vi "ex_getDaqmxChannelProperties.vi"(4 "error in (no error)":errorcluster, 5 "USI compliant names":bool, 6 "Number of channels (if no DAQmx task available)":i32, 7 "task":T4) -> (0 "error out":errorcluster, 1 "all properties":T1, 3 "channel properties":T2[][](array[typedef]))   [LabVIEW 2017]
uses:
  <vilib>/express/express shared/ex_EditUserDefinedProperties/ex_userdefproperties.ctl
  <vilib>/express/express shared/ExFile.llb/ex_userDefProperty.ctl
  <vilib>/express/express shared/ex_EditUserDefinedProperties/usiDataType.ctl
  <vilib>/express/express shared/ExFile.llb/ex_propertySource.ctl
  <vilib>/express/express shared/ExFile.llb/ex_TdmProperty.ctl
  <vilib>/express/express shared/ExFile.llb/ex_TdmData.ctl
panel:
  in  "File data":T1
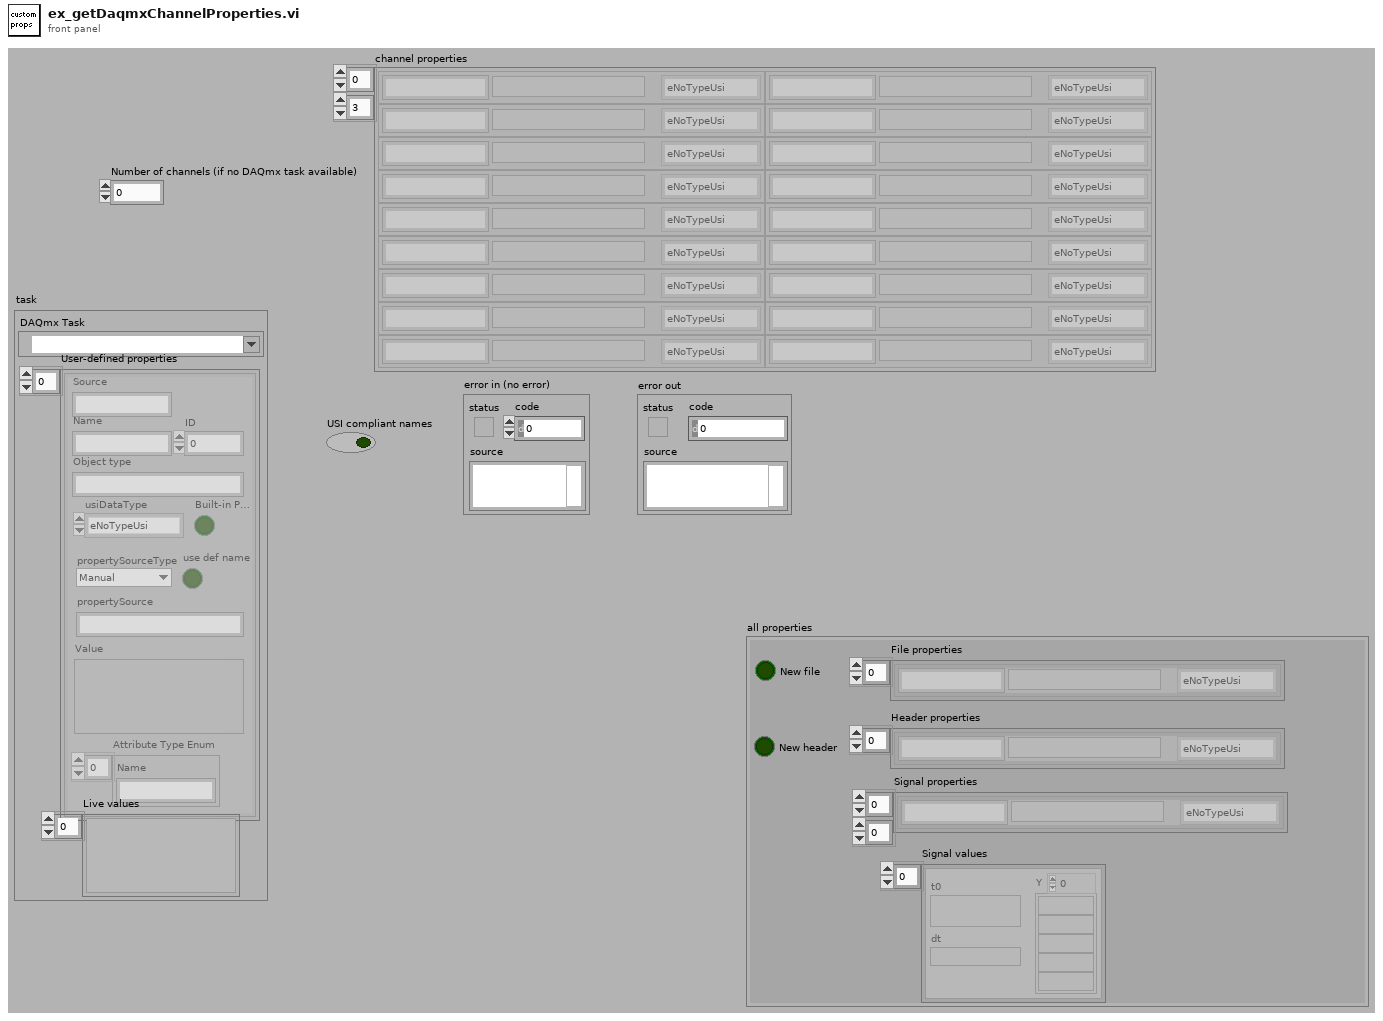
[diagram p1: front panel]
types:
  T1 = typedef "ex_TdmData.ctl" = cluster{"New file":bool, "New header":bool, "File properties":T2[], "Header properties":T2[], "Signal properties":T2[][], "Signal values":waveform(dbl)[]}
  T2 = typedef "ex_TdmProperty.ctl" = cluster{"Name":string, "Type":T3, "Value":variant}
  T3 = typedef "usiDataType.ctl" = enum16{"eNoTypeUsi", "eInt8Usi", "eInt16Usi", "eInt32Usi", "eInt64Usi", "eUInt8Usi", "eUInt16Usi", "eUInt32Usi", "eUInt64Usi", "eFloat32Usi", "eFloat64Usi", "- 0", "- 1", "- 2", "- 3", "- 4", "- 5", "- 6", "- 7", "- 8", "- 9", "eString8Usi", "eString16Usi", "eStringUsi", "eEnumUsi", "- 10", "- 11", "- 12", "- 13", "- 14", "eTimeUsi", "- 15", "- 16", "- 17", "- 18", "- 19", "- 20", "- 21", "- 22", "- 23", "eInstanceUsi", "eStoreUsi"}
  T4 = typedef "ex_userdefproperties.ctl" = cluster{"DAQmx Task":refnum<k21>, "User-defined properties":T5[], "Live values":variant[]}
  T5 = typedef "ex_userDefProperty.ctl" = cluster{"Name":string, "Object type":string, "usiDataType":T3, "propertySourceType":T6, "propertySource":string, "Value":variant, "ID":i32, "use def name":bool, "Source":string, "Built-in Prop":bool, "Attribute Type Enum":string[]}
  T6 = typedef "ex_propertySource.ctl" = enum16{"Manual", "System", "DAQmx Channel", "Terminal", "Ignore"}
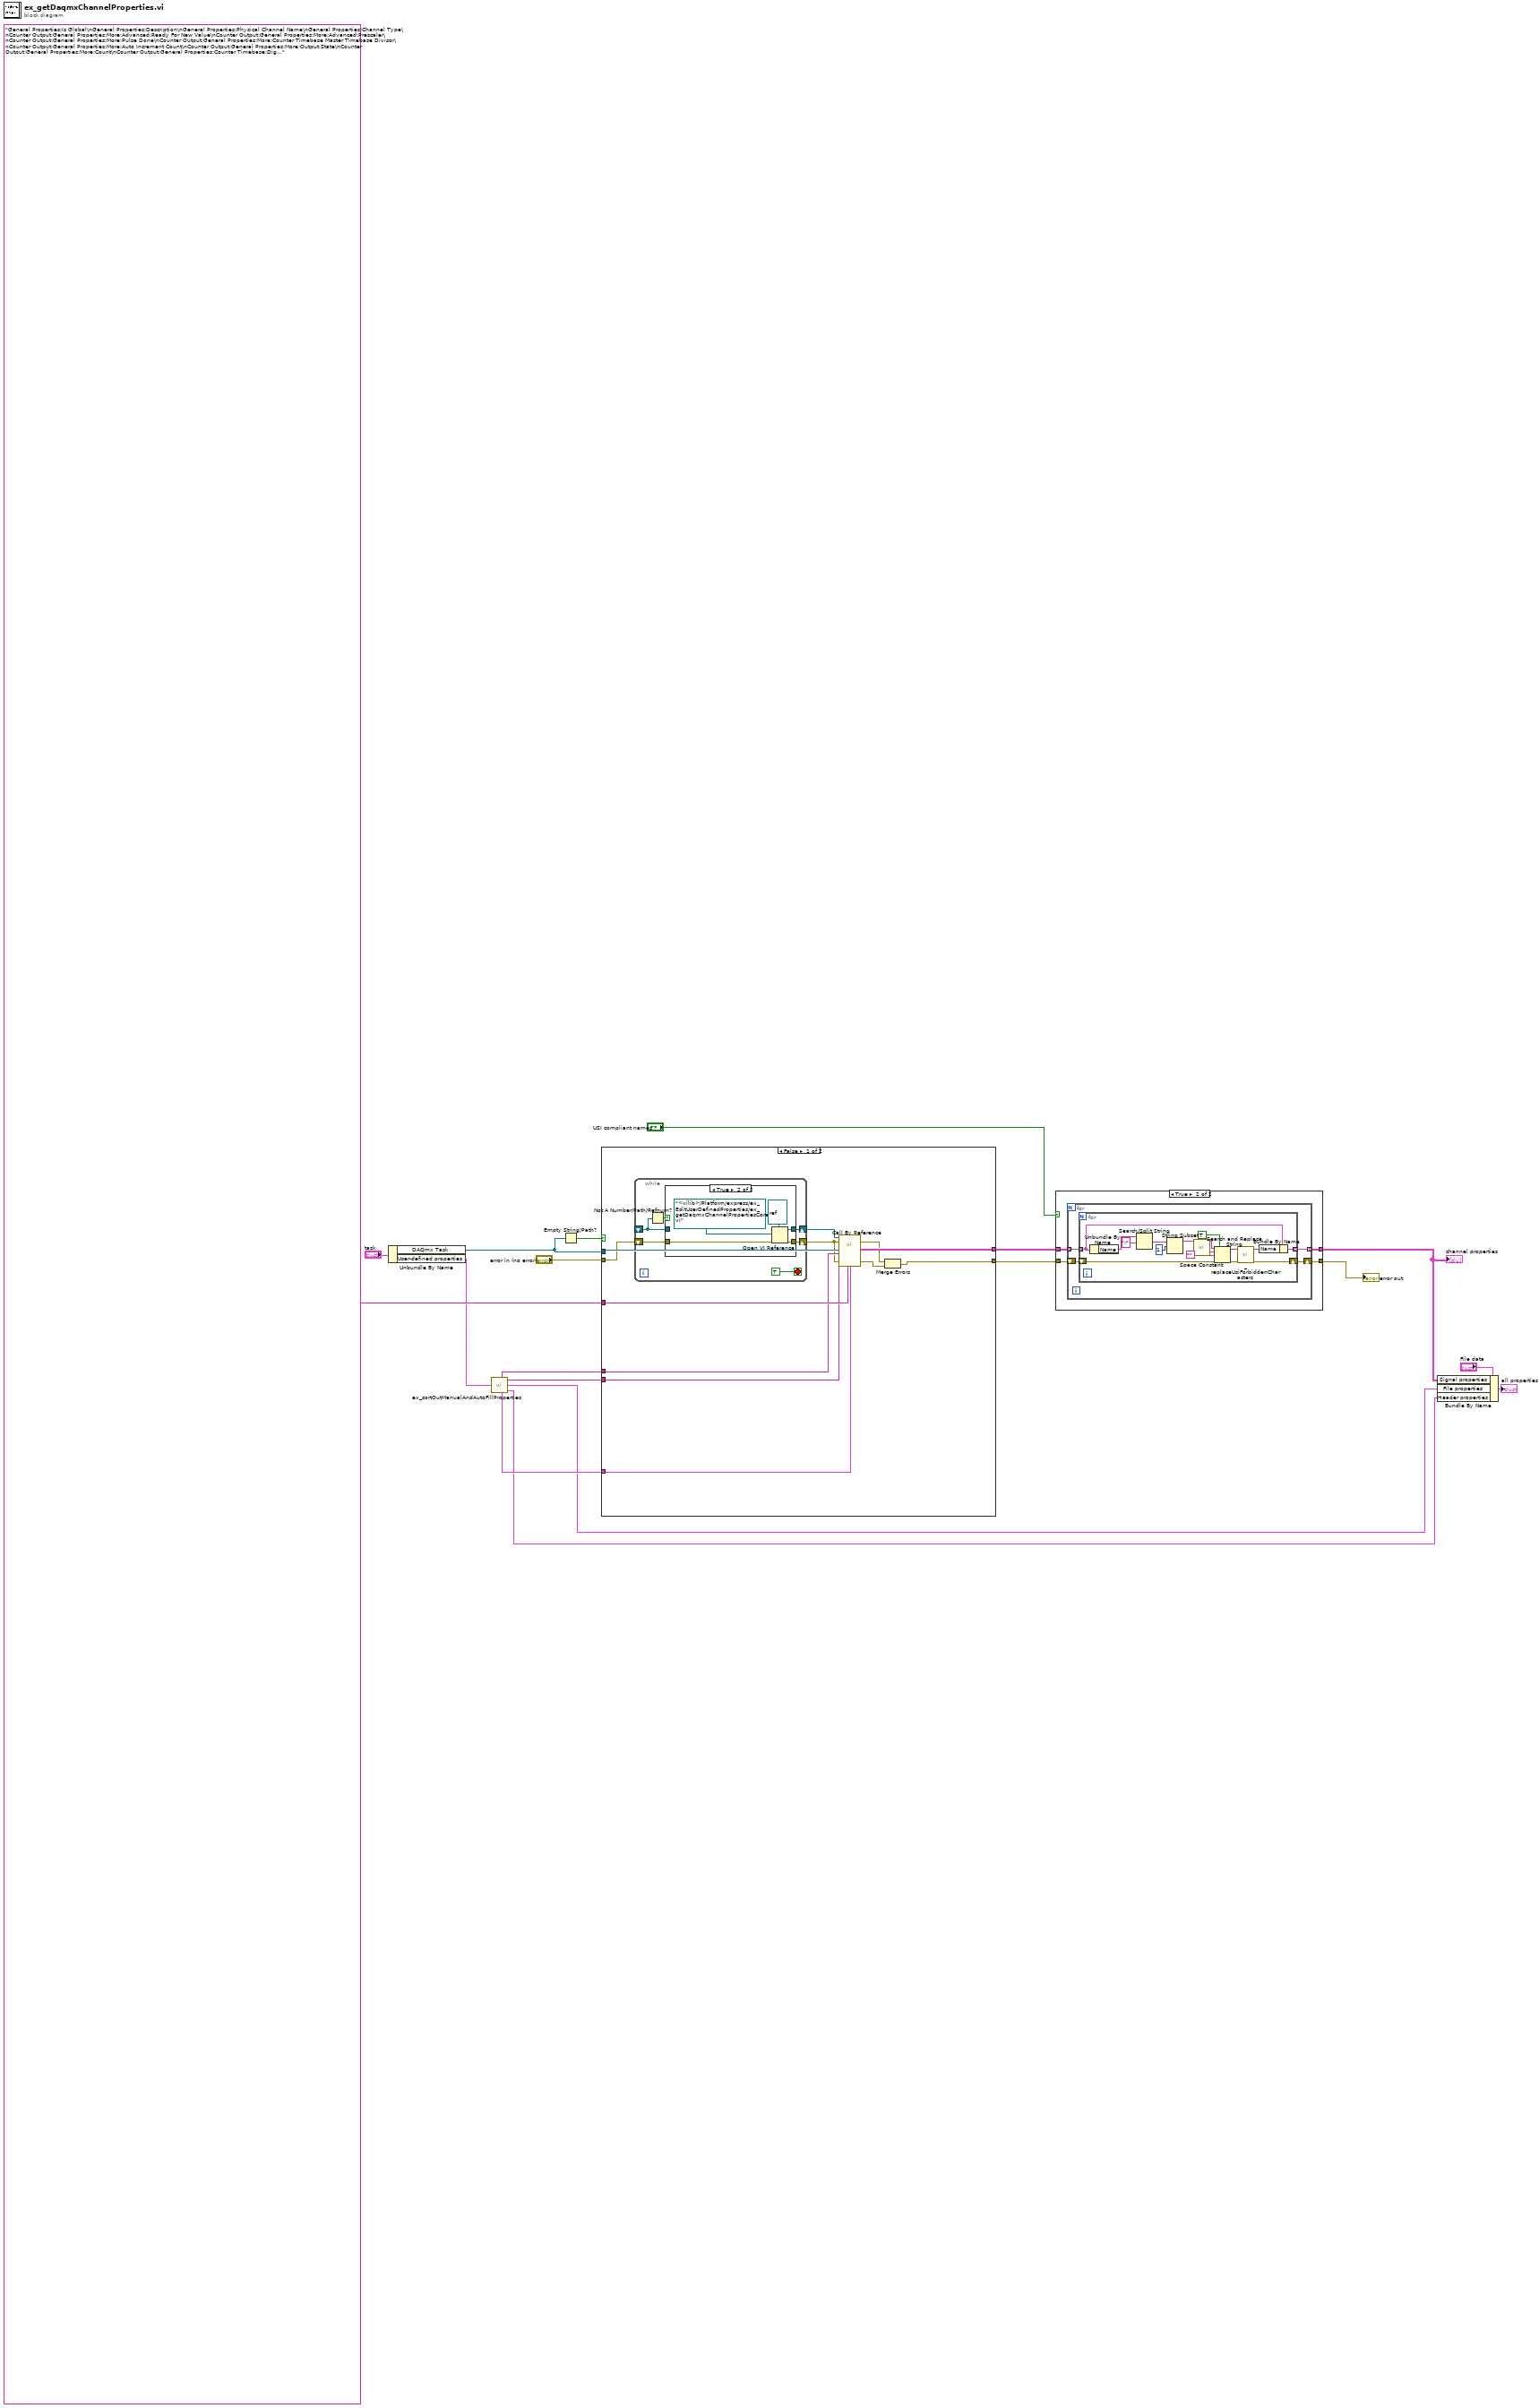
[diagram p0: block diagram]
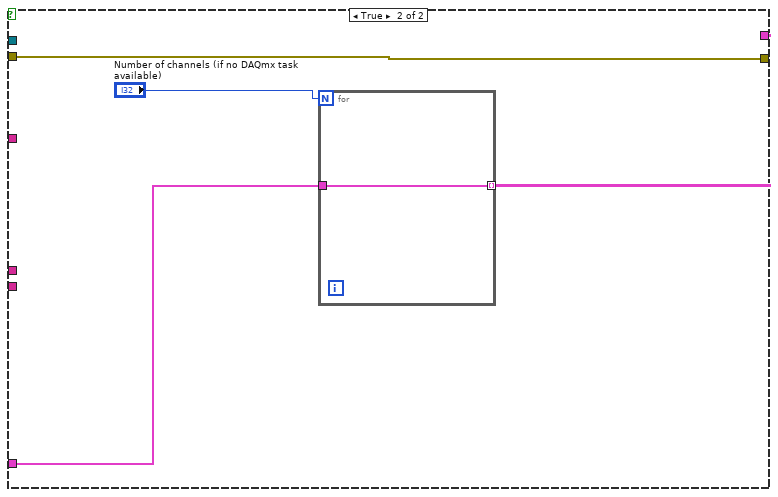
[diagram p3: hidden frame]
diagram:
  n1 = Unbundle By Name("task") -> ("DAQmx Task"=w2:refnum<k21>, "User-defined properties"=w13:T5[])
  n2 = call <vilib>:"ex_sortOutManualAndAutoFillProperties.vi"("User-defined properties"=w13) -> ("channelgroup props"=w6:T2[], "channel props"=w10:T2[], "file props"=w7:T2[], "property names (manual)"=w12:string[], "property names (autofill)"=w11:string[])
  n3 = Empty String/Path?(string/path=w2) -> (empty?=w1:bool)
  n4 = case shown="False" w1 {
    tunnel: "General Properties:Is Global\nGeneral Properties:Description\nGeneral Properties:Physical Channel Name\nGeneral Properties:Channel Type\nCounter Output:General Properties:More:Advanced:Ready For New Value\nCounter Output:General Properties:More:Advanced:Prescaler\nCounter Output:General Properties:More:Pulse Done\nCounter Output:General Properties:More:Counter Timebase Master Timebase Divisor\nCounter Output:General Properties:More:Auto Increment Count\nCounter Output:General Properties:More:Output State\nCounter Output:General Properties:More:Count\nCounter Output:General Properties:Counter Timebase:Digital Synchronization:Enable\nCounter Output:General Properties:Counter Timebase:Digital Filter:Timebase:Rate\nCounter Output:General Properties:Counter Timebase:Digital Filter:Timebase:Source\nCounter Output:General Properties:Counter Timebase:Digital Filter:Minimum Pulse Width\nCounter Output:General Properties:Counter Timebase:Digital Filter:Enable\nCounter Output:General Properties:Counter Timebase:Active Edge\nCounter Output:General Properties:Counter Timebase:Rate\nCounter Output:General Properties:Counter Timebase:Source\nCounter Output:Pulse:Ticks:Initial Delay\nCounter Output:Pulse:Ticks:Low Ticks\nCounter Output:Pulse:Ticks:High Ticks\nCounter Output:Pulse:Frequency:Initial Delay\nCounter Output:Pulse:Frequency:Frequency\nCounter Output:Pulse:Frequency:Units\nCounter Output:Pulse:Frequency:Duty Cycle\nCounter Output:Pulse:Time:Initial Delay\nCounter Output:Pulse:Time:Low Time\nCounter Output:Pulse:Time:High Time\nCounter Output:Pulse:Time:Units\nCounter Output:Pulse:Output Terminal\nCounter Output:Pulse:Idle State\nCounter Output:Output Type\nCounter Input:General Properties:More:Advanced:Prescaler\nCounter Input:General Properties:More:Advanced:Duplicate Count Prevention\nCounter Input:General Properties:More:Advanced:Data Transfer and Memory:Number Of Possibly Invalid Samples\nCounter Input:General Properties:More:Advanced:Data Transfer and Memory:Data Transfer Mechanism\nCounter Input:General Properties:More:Counter Timebase Master Timebase Divisor\nCounter Input:General Properties:More:Terminal Count Reached\nCounter Input:General Properties:More:Output State\nCounter Input:General Properties:More:Count\nCounter Input:General Properties:Counter Timebase:Digital Synchronization:Enable\nCounter Input:General Properties:Counter Timebase:Digital Filter:Timebase:Rate\nCounter Input:General Properties:Counter Timebase:Digital Filter:Timebase:Source\nCounter Input:General Properties:Counter Timebase:Digital Filter:Minimum Pulse Width\nCounter Input:General Properties:Counter Timebase:Digital Filter:Enable\nCounter Input:General Properties:Counter Timebase:Active Edge\nCounter Input:General Properties:Counter Timebase:Rate\nCounter Input:General Properties:Counter Timebase:Source\nCounter Input:Timestamp:GPS:Synchronization Source\nCounter Input:Timestamp:GPS:Synchronization Method\nCounter Input:Timestamp:Initial Seconds\nCounter Input:Timestamp:Units\nCounter Input:Semi-Period:Digital Synchronization:Enable\nCounter Input:Semi-Period:Digital Filter:Timebase:Rate\nCounter Input:Semi-Period:Digital Filter:Timebase:Source\nCounter Input:Semi-Period:Digital Filter:Minimum Pulse Width\nCounter Input:Semi-Period:Digital Filter:Enable\nCounter Input:Semi-Period:Starting Edge\nCounter Input:Semi-Period:Input Terminal\nCounter Input:Semi-Period:Units\nCounter Input:Two Edge Separation:Second:Digital Synchronization:Enable\nCounter Input:Two Edge Separation:Second:Digital Filter:Timebase:Rate\nCounter Input:Two Edge Separation:Second:Digital Filter:Timebase:Source\nCounter Input:Two Edge Separation:Second:Digital Filter:Minimum Pulse Width\nCounter Input:Two Edge Separation:Second:Digital Filter:Enable\nCounter Input:Two Edge Separation:Second:Edge\nCounter Input:Two Edge Separation:Second:Input Terminal\nCounter Input:Two Edge Separation:First:Digital Synchronization:Enable\nCounter Input:Two Edge Separation:First:Digital Filter:Timebase:Rate\nCounter Input:Two Edge Separation:First:Digital Filter:Timebase:Source\nCounter Input:Two Edge Separation:First:Digital Filter:Minimum Pulse Width\nCounter Input:Two Edge Separation:First:Digital Filter:Enable\nCounter Input:Two Edge Separation:First:Edge\nCounter Input:Two Edge Separation:First:Input Terminal\nCounter Input:Two Edge Separation:Units\nCounter Input:Pulse Width:Digital Synchronization:Enable\nCounter Input:Pulse Width:Digital Filter:Timebase:Rate\nCounter Input:Pulse Width:Digital Filter:Timebase:Source\nCounter Input:Pulse Width:Digital Filter:Minimum Pulse Width\nCounter Input:Pulse Width:Digital Filter:Enable\nCounter Input:Pulse Width:Starting Edge\nCounter Input:Pulse Width:Input Terminal\nCounter Input:Pulse Width:Units\nCounter Input:Position:Z Index Phase\nCounter Input:Position:Z Index Value\nCounter Input:Position:Z Index Enable\nCounter Input:Position:Z Input:Digital Synchronization:Enable\nCounter Input:Position:Z Input:Digital Filter:Timebase:Rate\nCounter Input:Position:Z Input:Digital Filter:Timebase:Source\nCounter Input:Position:Z Input:Digital Filter:Minimum Pulse Width\nCounter Input:Position:Z Input:Digital Filter:Enable\nCounter Input:Position:Z Input:Terminal\nCounter Input:Position:B Input:Digital Synchronization:Enable\nCounter Input:Position:B Input:Digital Filter:Timebase:Rate\nCounter Input:Position:B Input:Digital Filter:Timebase:Source\nCounter Input:Position:B Input:Digital Filter:Minimum Pulse Width\nCounter Input:Position:B Input:Digital Filter:Enable\nCounter Input:Position:B Input:Terminal\nCounter Input:Position:A Input:Digital Synchronization:Enable\nCounter Input:Position:A Input:Digital Filter:Timebase:Rate\nCounter Input:Position:A Input:Digital Filter:Timebase:Source\nCounter Input:Position:A Input:Digital Filter:Minimum Pulse Width\nCounter Input:Position:A Input:Digital Filter:Enable\nCounter Input:Position:A Input:Terminal\nCounter Input:Position:Decoding Type\nCounter Input:Position:Linear Encoder:Initial Position\nCounter Input:Position:Linear Encoder:Distance Per Pulse\nCounter Input:Position:Linear Encoder:Units\nCounter Input:Position:Angular Encoder:Initial Angle\nCounter Input:Position:Angular Encoder:Pulses Per Revolution\nCounter Input:Position:Angular Encoder:Units\nCounter Input:Count Edges:Digital Synchronization:Enable\nCounter Input:Count Edges:Digital Filter:Timebase:Rate\nCounter Input:Count Edges:Digital Filter:Timebase:Source\nCounter Input:Count Edges:Digital Filter:Minimum Pulse Width\nCounter Input:Count Edges:Digital Filter:Enable\nCounter Input:Count Edges:Active Edge\nCounter Input:Count Edges:Initial Count\nCounter Input:Count Edges:Count Direction:Digital Synchronization:Enable\nCounter Input:Count Edges:Count Direction:Digital Filter:Timebase:Rate\nCounter Input:Count Edges:Count Direction:Digital Filter:Timebase:Source\nCounter Input:Count Edges:Count Direction:Digital Filter:Minimum Pulse Width\nCounter Input:Count Edges:Count Direction:Digital Filter:Enable\nCounter Input:Count Edges:Count Direction:Terminal\nCounter Input:Count Edges:Count Direction:Direction\nCounter Input:Count Edges:Input Terminal\nCounter Input:Period:Digital Synchronization:Enable\nCounter Input:Period:Digital Filter:Timebase:Rate\nCounter Input:Period:Digital Filter:Timebase:Source\nCounter Input:Period:Digital Filter:Minimum Pulse Width\nCounter Input:Period:Digital Filter:Enable\nCounter Input:Period:Measurement Specifications:Large Range:Divisor\nCounter Input:Period:Measurement Specifications:High Frequency:Measurement Time\nCounter Input:Period:Measurement Specifications:Method\nCounter Input:Period:Starting Edge\nCounter Input:Period:Input Terminal\nCounter Input:Period:Units\nCounter Input:Frequency:Digital Synchronization:Enable\nCounter Input:Frequency:Digital Filter:Timebase:Rate\nCounter Input:Frequency:Digital Filter:Timebase:Source\nCounter Input:Frequency:Digital Filter:Minimum Pulse Width\nCounter Input:Frequency:Digital Filter:Enable\nCounter Input:Frequency:Measurement Specifications:Large Range:Divisor\nCounter Input:Frequency:Measurement Specifications:High Frequency:Measurement Time\nCounter Input:Frequency:Measurement Specifications:Method\nCounter Input:Frequency:Starting Edge\nCounter Input:Frequency:Input Terminal\nCounter Input:Frequency:Units\nCounter Input:Measurement Type\nCounter Input:Custom Scale Name\nCounter Input:Minimum Value\nCounter Input:Maximum Value\nDigital Output:General Properties:Advanced:Data Transfer and Memory:Data Transfer Request Condition\nDigital Output:General Properties:Advanced:Data Transfer and Memory:Data Transfer Mechanism\nDigital Output:General Properties:Advanced:Data Transfer and Memory:Use Only Onboard Memory\nDigital Output:Tristate\nDigital Output:Number of Lines\nDigital Output:Invert Lines\nDigital Output:Output Drive Type\nDigital Input:General Properties:Advanced:Data Transfer and Memory:Data Transfer Request Condition\nDigital Input:General Properties:Advanced:Data Transfer and Memory:Data Transfer Mechanism\nDigital Input:Tristate\nDigital Input:Digital Filter:Minimum Pulse Width\nDigital Input:Digital Filter:Enable\nDigital Input:Number of Lines\nDigital Input:Invert Lines\nAnalog Output:General Properties:Advanced:Enhanced Image Rejection Enable\nAnalog Output:General Properties:Advanced:Device Scaling Coefficients:Device Scaling Coefficients\nAnalog Output:General Properties:Advanced:Data Transfer and Memory:Memory Mapping for Programmed IO Enable\nAnalog Output:General Properties:Advanced:Data Transfer and Memory:Data Transfer Request Condition\nAnalog Output:General Properties:Advanced:Data Transfer and Memory:Data Transfer Mechanism\nAnalog Output:General Properties:Advanced:Data Transfer and Memory:Use Only Onboard Memory\nAnalog Output:General Properties:Advanced:Gain:Gain Value\nAnalog Output:General Properties:DAC:Reglitching Enable\nAnalog Output:General Properties:DAC:Offset Voltage:Value\nAnalog Output:General Properties:DAC:Offset Voltage:External Source\nAnalog Output:General Properties:DAC:Offset Voltage:Source\nAnalog Output:General Properties:DAC:Reference Voltage:Value\nAnalog Output:General Properties:DAC:Reference Voltage:External Source\nAnalog Output:General Properties:DAC:Reference Voltage:Source\nAnalog Output:General Properties:DAC:Reference Voltage:Allow Connecting DAC Reference to Ground at Runtime\nAnalog Output:General Properties:DAC:Reference Voltage:Connect DAC Reference to Ground\nAnalog Output:General Properties:DAC:Range:Low\nAnalog Output:General Properties:DAC:Range:High\nAnalog Output:General Properties:DAC:Resolution Value\nAnalog Output:General Properties:DAC:Resolution Units\nAnalog Output:General Properties:Output Configuration:Terminal Configuration\nAnalog Output:General Properties:Output Configuration:Idle Output Behavior\nAnalog Output:General Properties:Output Configuration:Load Impedance\nAnalog Output:General Properties:Output Configuration:Output Impedance\nAnalog Output:Current:Units\nAnalog Output:Voltage:Units\nAnalog Output:Output Type\nAnalog Output:Custom Scale Name\nAnalog Output:Minimum Value\nAnalog Output:Maximum Value\nAnalog Input:General Properties:Advanced:Enhanced Alias Rejection Enable\nAnalog Input:General Properties:Advanced:Device Scaling Coefficients:Device Scaling Coefficients\nAnalog Input:General Properties:Advanced:Data Transfer and Memory:Compression:Lossy LSB Removal:Compressed Sample Size\nAnalog Input:General Properties:Advanced:Data Transfer and Memory:Compression:Raw Data Compression Type\nAnalog Input:General Properties:Advanced:Data Transfer and Memory:Memory Mapping for Programmed IO Enable\nAnalog Input:General Properties:Advanced:Data Transfer and Memory:Data Transfer Custom Threshold\nAnalog Input:General Properties:Advanced:Data Transfer and Memory:Data Transfer Request Condition\nAnalog Input:General Properties:Advanced:Data Transfer and Memory:Data Transfer Mechanism\nAnalog Input:General Properties:Advanced:High Accuracy Settings:Auto Zero Mode\nAnalog Input:General Properties:Advanced:Sample and Hold Enable\nAnalog Input:General Properties:Advanced:Gain:Gain Value\nAnalog Input:General Properties:Advanced:Range:Low\nAnalog Input:General Properties:Advanced:Range:High\nAnalog Input:General Properties:Channel Calibration:Verification:Acquired Values\nAnalog Input:General Properties:Channel Calibration:Verification:Reference Values\nAnalog Input:General Properties:Channel Calibration:Description\nAnalog Input:General Properties:Channel Calibration:Operator Name\nAnalog Input:General Properties:Channel Calibration:Scaling Parameters:Polynomial:Reverse Coefficients\nAnalog Input:General Properties:Channel Calibration:Scaling Parameters:Polynomial:Forward Coefficients\nAnalog Input:General Properties:Channel Calibration:Scaling Parameters:Table:Scaled Values\nAnalog Input:General Properties:Channel Calibration:Scaling Parameters:Table:Pre-Scaled Values\nAnalog Input:General Properties:Channel Calibration:Scaling Parameters:Scale Type\nAnalog Input:General Properties:Channel Calibration:Expiration Date\nAnalog Input:General Properties:Channel Calibration:Calibration Date\nAnalog Input:General Properties:Channel Calibration:Apply Calibration If Expired\nAnalog Input:General Properties:Channel Calibration:Enable Calibration\nAnalog Input:General Properties:Channel Calibration:Has Valid Calibration Information\nAnalog Input:General Properties:Digitizer/ADC:Dither:Enable\nAnalog Input:General Properties:Digitizer/ADC:Raw Sample Justification\nAnalog Input:General Properties:Digitizer/ADC:Raw Sample Size\nAnalog Input:General Properties:Digitizer/ADC:Resolution Value\nAnalog Input:General Properties:Digitizer/ADC:Resolution Units\nAnalog Input:General Properties:Filter:Analog Lowpass:Advanced:Switched Capacitor:Output Clock Divisor\nAnalog Input:General Properties:Filter:Analog Lowpass:Advanced:Switched Capacitor:External Clock Divisor\nAnalog Input:General Properties:Filter:Analog Lowpass:Advanced:Switched Capacitor:External Clock Frequency\nAnalog Input:General Properties:Filter:Analog Lowpass:Advanced:Switched Capacitor:Clock Source\nAnalog Input:General Properties:Filter:Analog Lowpass:Cutoff Frequency\nAnalog Input:General Properties:Filter:Analog Lowpass:Enable\nAnalog Input:General Properties:Signal Conditioning:Probe/Attenuator:Attenuation Value\nAnalog Input:General Properties:Signal Conditioning:Excitation:AC Excitation:Wire Mode\nAnalog Input:General Properties:Signal Conditioning:Excitation:AC Excitation:Synchronization Enable\nAnalog Input:General Properties:Signal Conditioning:Excitation:AC Excitation:Frequency\nAnalog Input:General Properties:Signal Conditioning:Excitation:Advanced:Voltage or Current\nAnalog Input:General Properties:Signal Conditioning:Excitation:Advanced:DC or AC\nAnalog Input:General Properties:Signal Conditioning:Excitation:Advanced:Actual Excitation Value\nAnalog Input:General Properties:Signal Conditioning:Excitation:Advanced:Use Multiplexed Excitation\nAnalog Input:General Properties:Signal Conditioning:Excitation:Advanced:Use Excitation For Scaling\nAnalog Input:General Properties:Signal Conditioning:Excitation:Value\nAnalog Input:General Properties:Signal Conditioning:Excitation:Source\nAnalog Input:General Properties:Signal Conditioning:Current Shunt Resistor:Value\nAnalog Input:General Properties:Signal Conditioning:Current Shunt Resistor:Location\nAnalog Input:General Properties:Signal Conditioning:Bridge:Balance:Fine Potentiometer\nAnalog Input:General Properties:Signal Conditioning:Bridge:Balance:Coarse Potentiometer\nAnalog Input:General Properties:Signal Conditioning:Bridge:Shunt Cal:Gain Adjustment\nAnalog Input:General Properties:Signal Conditioning:Bridge:Shunt Cal:Shunt Cal Select\nAnalog Input:General Properties:Signal Conditioning:Bridge:Shunt Cal:Shunt Cal Enable\nAnalog Input:General Properties:Signal Conditioning:Bridge:Initial Bridge Voltage\nAnalog Input:General Properties:Signal Conditioning:Bridge:Nominal Resistance\nAnalog Input:General Properties:Signal Conditioning:Bridge:Configuration\nAnalog Input:General Properties:Signal Conditioning:Lead Wire Resistance\nAnalog Input:General Properties:Signal Conditioning:Resistance Configuration\nAnalog Input:General Properties:Input Configuration:Input Source\nAnalog Input:General Properties:Input Configuration:Terminal Configuration\nAnalog Input:General Properties:Input Configuration:Impedance\nAnalog Input:General Properties:Input Configuration:Coupling\nAnalog Input:TEDS:Units\nAnalog Input:Acceleration:Accelerometer:Sensitivity Units\nAnalog Input:Acceleration:Accelerometer:Sensitivity\nAnalog Input:Acceleration:Units\nAnalog Input:Sound Pressure:Microphone:Sensitivity\nAnalog Input:Sound Pressure:Units\nAnalog Input:Sound Pressure:Maximum Sound Pressure Level\nAnalog Input:Position:RVDT:Sensitivity Units\nAnalog Input:Position:RVDT:Sensitivity\nAnalog Input:Position:RVDT:Units\nAnalog Input:Position:LVDT:Sensitivity Units\nAnalog Input:Position:LVDT:Sensitivity\nAnalog Input:Position:LVDT:Units\nAnalog Input:Frequency:Voltage:Hysteresis\nAnalog Input:Frequency:Voltage:Threshold Level\nAnalog Input:Frequency:Units\nAnalog Input:Resistance:Units\nAnalog Input:Strain:Strain Gage:Configuration\nAnalog Input:Strain:Strain Gage:Poisson Ratio\nAnalog Input:Strain:Strain Gage:Gage Factor\nAnalog Input:Strain:Units\nAnalog Input:Current:Units\nAnalog Input:Temperature:Advanced:Force Read from Channel\nAnalog Input:Temperature:Thermistor:R1\nAnalog Input:Temperature:Thermistor:C\nAnalog Input:Temperature:Thermistor:B\nAnalog Input:Temperature:Thermistor:A\nAnalog Input:Temperature:RTD:Custom:C\nAnalog Input:Temperature:RTD:Custom:B\nAnalog Input:Temperature:RTD:Custom:A\nAnalog Input:Temperature:RTD:R0\nAnalog Input:Temperature:RTD:Type\nAnalog Input:Temperature:Thermocouple:CJC Channel\nAnalog Input:Temperature:Thermocouple:CJC Value\nAnalog Input:Temperature:Thermocouple:CJC Source\nAnalog Input:Temperature:Thermocouple:Type\nAnalog Input:Temperature:Units\nAnalog Input:Voltage:Units\nAnalog Input:Measurement Type\nAnalog Input:Custom Scale Name\nAnalog Input:Minimum Value\nAnalog Input:Maximum Value\n" -> [w28 _]
    tunnel: "error in (no error)" -> [w23 w47]
    tunnel: w2 -> [w29 _]
    tunnel: w12 -> [w26 _]
    tunnel: w11 -> [w27 _]
    tunnel: w10 -> [w24 w45]
    tunnel: [w25 w44] -> w4
    tunnel: [w19 w47] -> w3
    frame False {
      n5 = while {
        shift-right: [w36] -> w30
        shift-left: _ -> [w31]
        shift-right: [w35] -> w22
        shift-left: w23 -> [w33]
        stop <- TRUE stop-if-true
        n6 = Not A Number/Path/Refnum?(number/path/refnum=w31) -> (NaN/Path/Refnum?=w32:bool)
        n7 = case shown="True" w32 {
          tunnel: [w37 w42] -> w36
          tunnel: [w38 w41] -> w35
          tunnel: w33 -> [w38 w39]
          tunnel: w31 -> [w37 _]
          frame False {
          }
          frame True {
            n8 = Open VI Reference(type specifier VI Refnum (for type only)=refnum<vi> refnum, vi path=path "<vilib>/Platform/express/ex_EditUserDefinedProperties/ex_getDaqmxChannelPropertiesCore.vi", error in (no error)=w39) -> (vi reference=w42:refnum<vi>, error out=w41:errorcluster)  [unwired: 3 out]
          }
        }
      }
      n9 = call-by-ref "?"(reference=w30, error in=w22, "channel props"=w24, "String"=w28, 8:"error in (no error)"=w22, "property names (manual)"=w26, "property names (autofill)"=w27, "DAQmx Task"=w29) -> (error out=w21:errorcluster, 0:"error out"=w20:errorcluster, "Array"=w25:T2[][])  [unwired: 3 in, 2 out]
      n10 = Merge Errors(w21, w20) -> (w19:errorcluster)
    }
    frame True {
      n11 = for {
        N: "Number of channels (if no DAQmx task available)" -> [_]
        tunnel: w45 -> [w48]
        tunnel: [w48] -> w44 mode=indexing
      }
    }
  }
  n12 = case shown="True" "USI compliant names" {
    tunnel: w4 -> [w49 w54]
    tunnel: w3 -> [w50 w53]
    tunnel: [w50 w52] -> w16
    tunnel: [w49 w51] -> w8
    frame False {
    }
    frame True {
      n13 = for {
        tunnel: w54 -> [w58] mode=indexing
        shift-right: [w56] -> w52
        shift-left: w53 -> [w57]
        tunnel: [w55] -> w51 mode=indexing
        n14 = for {
          tunnel: w58 -> [w70] mode=indexing
          shift-right: [w60] -> w56
          shift-left: w57 -> [w71]
          tunnel: [w69] -> w55 mode=indexing
          n15 = Unbundle By Name(w70) -> ("Name"=w68:string)
          n16 = Search/Split String(string=w68, search string/char (-)=":" ("search string")) -> (match + rest of string=w65:string)  [unwired: 3 out]
          n17 = String Subset(string=w65, offset (0)=1) -> (substring=w67:string)  [unwired: 1 out]
          n18 = call <vilib>:"Space Constant.vi"() -> ("String"=w73:string)
          n19 = Search and Replace String(replace all?=TRUE ("replace all? (F)"), input string=w67, search string=w73, replace string="", error in=w71) -> (result string=w61:string, error out=w59:errorcluster)  [unwired: 5 out]
          n20 = call <vilib>:"_replaceUsiForbiddenCharacters.vi"("error in (no error)"=w59, "string in"=w61) -> ("error out"=w60:errorcluster, "string out"=w63:string)  [unwired: 1 in, 3 out]
          n21 = Bundle By Name(cluster=w70, "Name"=w63) -> (w69:T2)
        }
      }
    }
  }
  "channel properties" <- w8
  "error out" <- w16
  n22 = Bundle By Name(cluster="File data", "Signal properties"=w8, "File properties"=w7, "Header properties"=w6) -> (→"all properties":T1)
